vi "ARTIQ-Client Submit Command.vi"(8 "error in (no error)":errorcluster, 11 "Kasli Wrapper 2.0 in":refnum<class "Kasli Wrapper 2.0.lvclass">) -> (0 "error out":errorcluster, 2 "artiq-client submit":string, 3 "Kasli Wrapper 2.0 out":refnum<class "Kasli Wrapper 2.0.lvclass">)   [LabVIEW 2020, in "Kasli Wrapper 2.0.lvlib" / "Kasli Wrapper 2.0.lvclass"]
uses:
  Kasli Wrapper 2.0.lvclass
  Kasli Wrapper 2.0.lvclass/Kasli Wrapper 2.0.ctl
  Run Utilities/Run Instance/Run Instance.lvclass
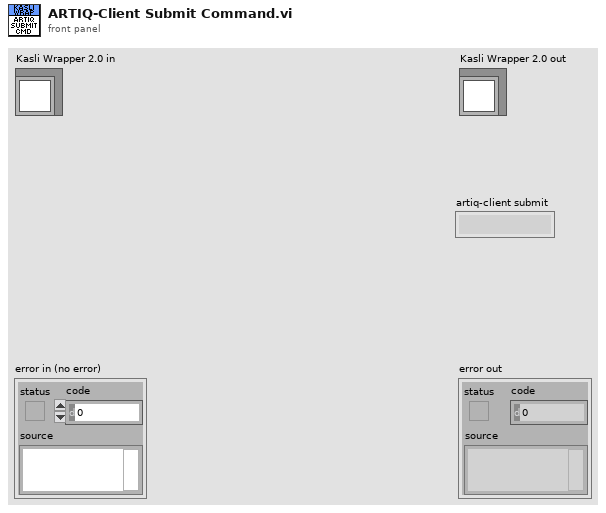
[diagram p1: front panel]
types:
  T1 = typedef "Run Utilities.lvlib/DAQ Control.ctl" = enum16{"On", "Off", "External"}
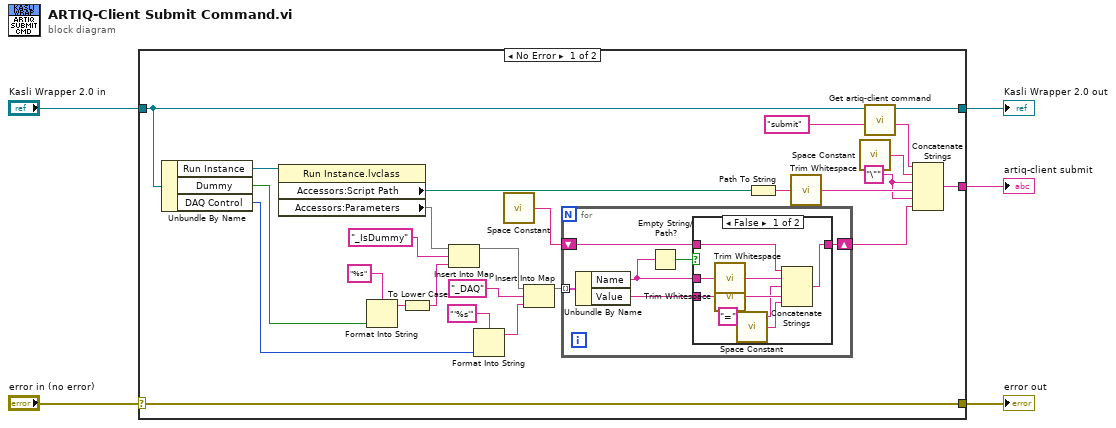
[diagram p0: block diagram]
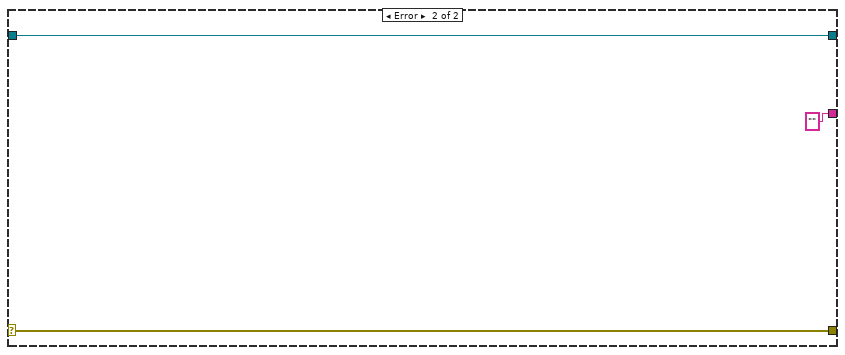
[diagram p3: hidden frame]
diagram:
  n1 = case shown="No Error" "error in (no error)" {
    selector: "error in (no error)" -> [w31 w49]
    tunnel: [w31 w49] -> w4
    tunnel: [w9 w48] -> w2
    tunnel: "Kasli Wrapper 2.0 in" -> [w10 w48]
    tunnel: [w12 ""] -> w1
    frame No Error {
      w28 = "\"" ("string")
      n2 = Unbundle By Name(w10) -> ("Run Instance"=w15:refnum<class "Run Instance.lvclass">, "Dummy"=w14:bool, "DAQ Control"=w13:T1)
      n3 = property class="Run Instance.lvclass"(reference=w15) -> ("Accessors:Script Path"=w27:path, "Accessors:Parameters"=w18:map{string, string})  [unwired: 1 in, 2 out]
      n4 = Format Into String(format string="%s", w14) -> (resulting string=w17:string)  [unwired: 2 in, 1 out]
      n5 = To Lower Case(string=w17) -> (all lower case string=w16:string)
      n6 = Insert Into Map(map in=w18, key="_IsDummy", value=w16) -> (map out=w22:map{string, string})  [unwired: 2 out]
      n7 = Format Into String(format string="'%s'", w13) -> (resulting string=w20:string)  [unwired: 2 in, 1 out]
      n8 = call <vilib>:"Space Constant.vi"() -> ("String"=w26:string)
      n9 = Insert Into Map(map in=w22, key="_DAQ", value=w20) -> (map out=w21:map{string, string})  [unwired: 2 out]
      n10 = for {
        shift-right: [w35] -> w7
        shift-left: w26 -> [w36]
        tunnel: w21 -> [w34] mode=indexing
        n11 = Unbundle By Name(w34) -> ("Name"=w32:string, "Value"=w33:string)
        n12 = Empty String/Path?(string/path=w32) -> (empty?=w37:bool)
        n13 = case shown="False" w37 {
          tunnel: w32 -> [w39 _]
          tunnel: w33 -> [w38 _]
          tunnel: w36 -> [w41 w46]
          tunnel: [w40 w46] -> w35
          frame False {
            n14 = call <vilib>:"Trim Whitespace.vi"("string"=w39) -> ("trimmed string"=w45:string)  [unwired: 1 in]
            n15 = call <vilib>:"Trim Whitespace.vi"("string"=w38) -> ("trimmed string"=w44:string)  [unwired: 1 in]
            n16 = call <vilib>:"Space Constant.vi"() -> ("String"=w42:string)
            n17 = Concatenate Strings(w41, w45, "=" ("string"), w44, w42) -> (w40:string)
          }
          frame True {
          }
        }
      }
      n18 = Path To String(path=w27) -> (string=w30:string)
      n19 = call <vilib>:"Trim Whitespace.vi"("string"=w30) -> ("trimmed string"=w29:string)  [unwired: 1 in]
      n20 = call <vilib>:"Space Constant.vi"() -> ("String"=w8:string)
      n21 = call-dynamic "Get artiq-client command.vi"("sub-command"="submit" ("string"), "Kasli Wrapper 2.0 in"=w10) -> ("command"=w6:string, "Kasli Wrapper 2.0 out"=w9:refnum<class "Kasli Wrapper 2.0.lvclass">)  [unwired: 8 in]
      n22 = Concatenate Strings(w6, w8, w28, w29, w28, w7) -> (w12:string)
    }
    frame Error {
    }
  }
  "error out" <- w4
  "Kasli Wrapper 2.0 out" <- w2
  "artiq-client submit" <- w1
